vi "Add Module.vi"(8 "error in":errorcluster, 10 "module path":string, 11 "routing and faulting in":T1 format="%.0x") -> (0 "error out":errorcluster, 2 "unique module identifier":string, 3 "routing and faulting out":T1 format="%.0x")   [LabVIEW 2020, in "Routing and Faulting Scripting.lvlib"]
uses:
  Routing and Faulting Scripting.lvlib
  <vilib>/NI VeriStand/Custom Device API/Custom Device Item Ref.ctl
  NationalInstruments.VeriStand.SystemStorage
  Constants/Scripting Constants.vi
  Routing and Faulting Hardware API/Routing and Faulting Hardware API.lvlib
  <vilib>/NI VeriStand/Custom Device API/Custom Device API.lvlib
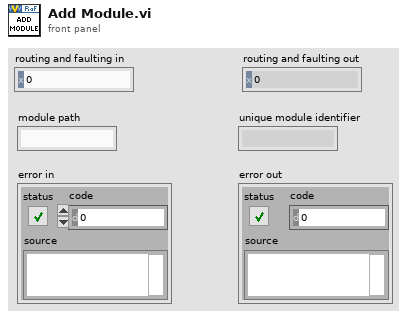
[diagram p1: front panel]
types:
  T1 = typedef "Custom Device API.lvlib/Custom Device Item Ref.ctl" = u64
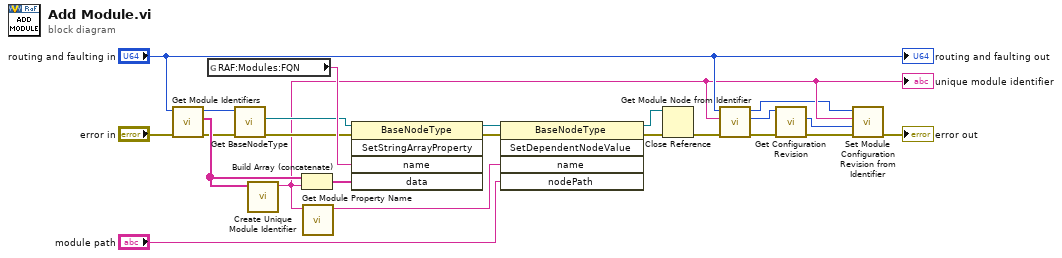
[diagram p0: block diagram]
diagram:
  n1 = call "Get Module Identifiers.vi"("error in"="error in", "routing and faulting in"="routing and faulting in") -> ("error out"=w16:errorcluster, "module Identifier"=w23:string[], "routing and faulting out"=w13:T1)  [unwired: 7 in]
  n2 = global read "Scripting Constants.vi" "RAF:Modules:FQN"() -> (w22:string)
  n3 = call "Get BaseNodeType.vi"("error in"=w16, "item in"=w13) -> ("error out"=w15:errorcluster, "BaseNodeType"=w14:refnum<k24>)  [unwired: 7 in, 1 out]
  n4 = call "Create Unique Module Identifier.vi"("existing module identifiers"=w23) -> ("unique module identifier"=w5:string)  [unwired: 10 in]
  "unique module identifier" <- w5
  n5 = Build Array (concatenate)(w23, w5) -> (w21:string[])
  n6 = call "Get Module Property Name.vi"("module identifier"=w5) -> ("module property name"=w12:string)  [unwired: 10 in]
  n7 = invoke class="BaseNodeType" method="SetStringArrayProperty"(reference=w14, error in=w15, "name"=w22, "data"=w21) -> (reference out=w18:refnum<k24>, error out=w19:errorcluster)  [unwired: 1 in, 3 out]
  n8 = invoke class="BaseNodeType" method="SetDependentNodeValue"(reference=w18, error in=w19, "name"=w12, "nodePath"="module path") -> (reference out=w6:refnum<k24>, error out=w11:errorcluster)  [unwired: 1 in, 3 out]
  n9 = Close Reference(reference=w6, error in (no error)=w11) -> (error out=w7:errorcluster)
  n10 = call "Get Module Node from Identifier.vi"("error in"=w7, "module identifier"=w5, "routing and faulting in"="routing and faulting in") -> ("error out"=w9:errorcluster, "module node"=w8:T1, "routing and faulting out"=w2:T1)  [unwired: 5 in, 1 out]
  n11 = call "Get Configuration Revision.vi"("error in (no error)"=w9, "Hardware Ref in"=w8) -> ("error out"=w4:errorcluster, "Configuration Revision"=w1:u32)  [unwired: 6 in, 2 out]
  n12 = call "Set Module Configuration Revision from Identifier.vi"("error in"=w4, "revision"=w1, "module identifier"=w5, "routing and faulting in"=w2) -> ("error out"=→"error out":errorcluster)  [unwired: 6 in, 1 out]
  "routing and faulting out" <- "routing and faulting in"
